vi "FIFO Flush-inter trial FIFO.vi"(8 "error in":errorcluster, 11 "FPGA VI Ref":T1) -> (0 "error out":errorcluster, 3 "FPGA VI Reference Out":T1)   [LabVIEW 2017]
uses:
  RIG-SPECIFIC FILES/FPGA Refs/FPGA Ref.ctl
  <vilib>/Utility/error.llb/Error Cluster From Error Code.vi
  <vilib>/rvi/errors/niLvFpgaAdjustHostInterfaceError.vi
  <vilib>/rvi/interface/nirviMethod/nirviMethod.xnode
  <vilib>/FPGAPlugInAG/Dynamic/niLvFpga_ReadFifo_Dynamic.vi
  <vilib>/rvi/errors/niLvFpgaMergeErrorWithErrorCode.vi
panel:
  in  "Manual force stop":bool
  out "Data Inter trial Time":u64[](array[numeric])
  out "Inter trial time zero":u32
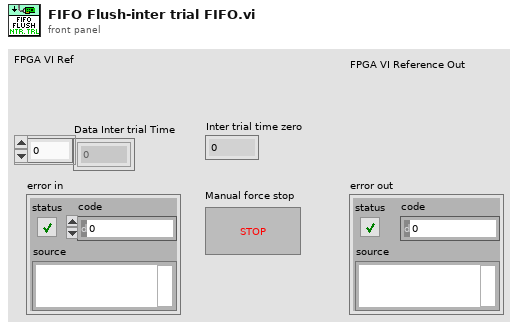
[diagram p1: front panel]
types:
  T1 = typedef "FPGA Ref.ctl" = refnum<k20>
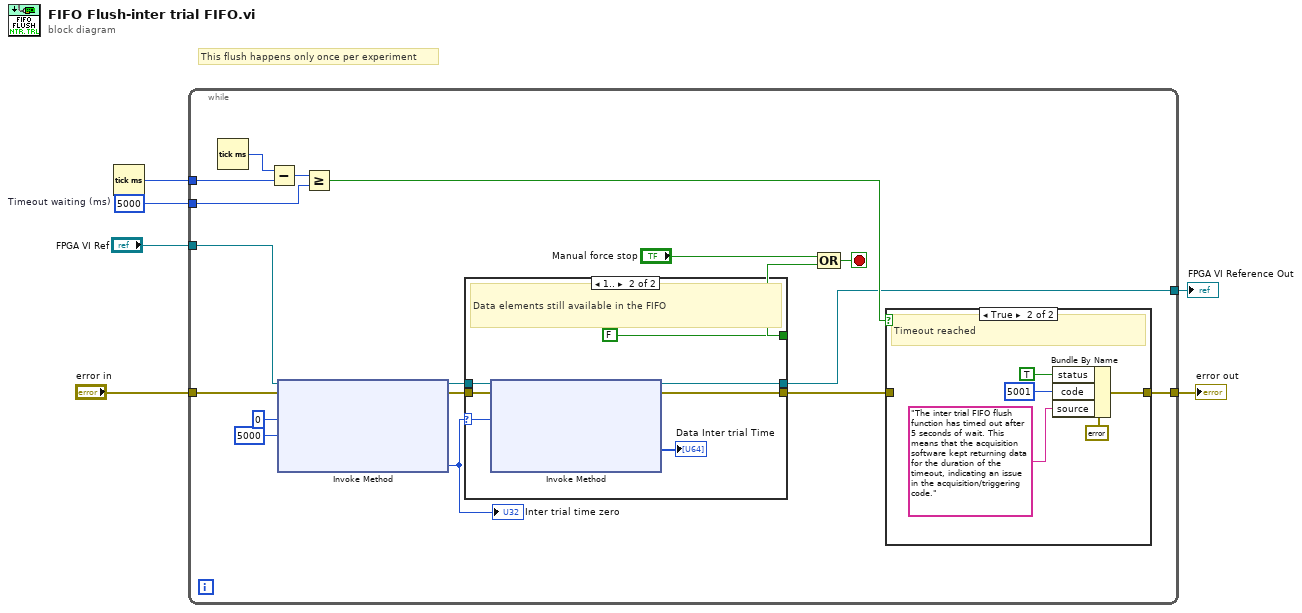
[diagram p0: block diagram]
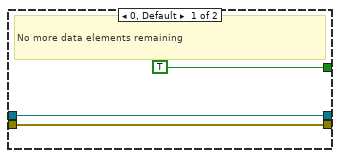
[diagram p2: hidden frame]
diagram:
  w5 = u32 5000  # Timeout waiting (ms)
  # "This flush happens only once per experiment"
  n1 = Tick Count (ms)() -> (millisecond timer value=w6:u32)
  n2 = while {
    tunnel: w6 -> [w21]
    tunnel: w5 -> [w22]
    tunnel: "FPGA VI Ref" -> [w14]
    tunnel: "error in" -> [w13]
    tunnel: [w8] -> w2
    tunnel: [w7] -> w1
    stop <- w11 stop-if-true
    n3 = Tick Count (ms)() -> (millisecond timer value=w24:u32)
    n4 = Subtract(x=w24, y=w21) -> (x-y=w23:u32)
    n5 = xnode "Invoke Method"("FPGA VI Reference In"=w14, "error in"=w13, "Number of Elements"=u32 0, "Timeout (ms)"=5000) -> ("FPGA VI Reference Out"=w16:T1, "error out"=w15:errorcluster, "Elements Remaining"=w19:u32)  [unwired: 1 out]
    "Inter trial time zero" <- w19
    n6 = Greater Or Equal?(x=w23, y=w22) -> (x >= y?=w20:bool)
    n7 = case shown="1.." w19 {
      selector: w19 -> [_ w31]
      tunnel: w15 -> [w26 w34]
      tunnel: w16 -> [w25 w33]
      tunnel: [w26 w32] -> w9
      tunnel: [TRUE FALSE] -> w10
      tunnel: [w25 w28] -> w7
      frame 0, Default {
        # "No more data elements remaining"
      }
      frame 1.. {
        # "Data elements still available in the FIFO"
        n8 = xnode "Invoke Method"("FPGA VI Reference In"=w33, "error in"=w34, "Number of Elements"=w31) -> ("FPGA VI Reference Out"=w28:T1, "error out"=w32:errorcluster, "Data"=→"Data Inter trial Time":u64[])  [unwired: 1 in, 1 out]
      }
    }
    n9 = Compound Arithmetic op=OR("Manual force stop", w10) -> (w11:bool)
    n10 = case shown="True" w20 {
      tunnel: [w35 w36] -> w8
      tunnel: w9 -> [w35 _]
      frame False {
      }
      frame True {
        # "Timeout reached"
        n11 = Bundle By Name(cluster=errorcluster {"status"=TRUE, "code"=5001, "source"=""} ("error out"), "status"=TRUE, "code"=5001, "source"="The inter trial FIFO flush function has timed out after 5 seconds of wait. This means that the acquisition software kept returning data for the duration of the timeout, indicating an issue in the acquisition/triggering code." ("Error Source")) -> (w36:errorcluster)
      }
    }
  }
  "error out" <- w2
  "FPGA VI Reference Out" <- w1
